vi "rtin_setControlMoveGPIO.vi"(8 "error":errorcluster, 9 "enable":bool=TRUE, 10 "axis":i32, 11 "connection ID":refnum<k5>) -> (0 "error out":errorcluster, 2 "axis_out":i32, 3 "connection ID out":refnum<k5>)   [LabVIEW 2016, in "amc_api.lvlib"]
doc: "This function sets the status for real time input on the selected axis in closed-loop mode."
uses:
  amc_api.lvlib
panel:
  out "jsonRespIn":string
  out "JSON-response":string="{\"jsonrpc\":\"2.0\",\"method\":\"\",\"params\":[5,1.245,true,\"name\"],\"id\":\"1\"}"
  out "JSON request":string
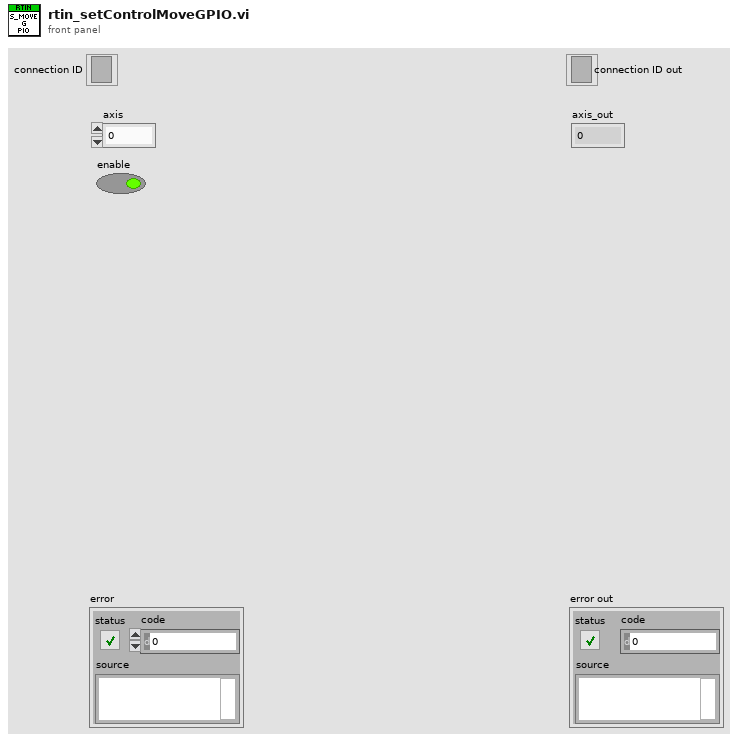
[diagram p1: front panel]
types:
  T1 = cluster{"jsonrpc":string, "method":string, "params":string[], "id":string, "api":i32, "pid":string}
  T2 = enum16{"Standard", "Buffered", "CRLF", "Immediate"}
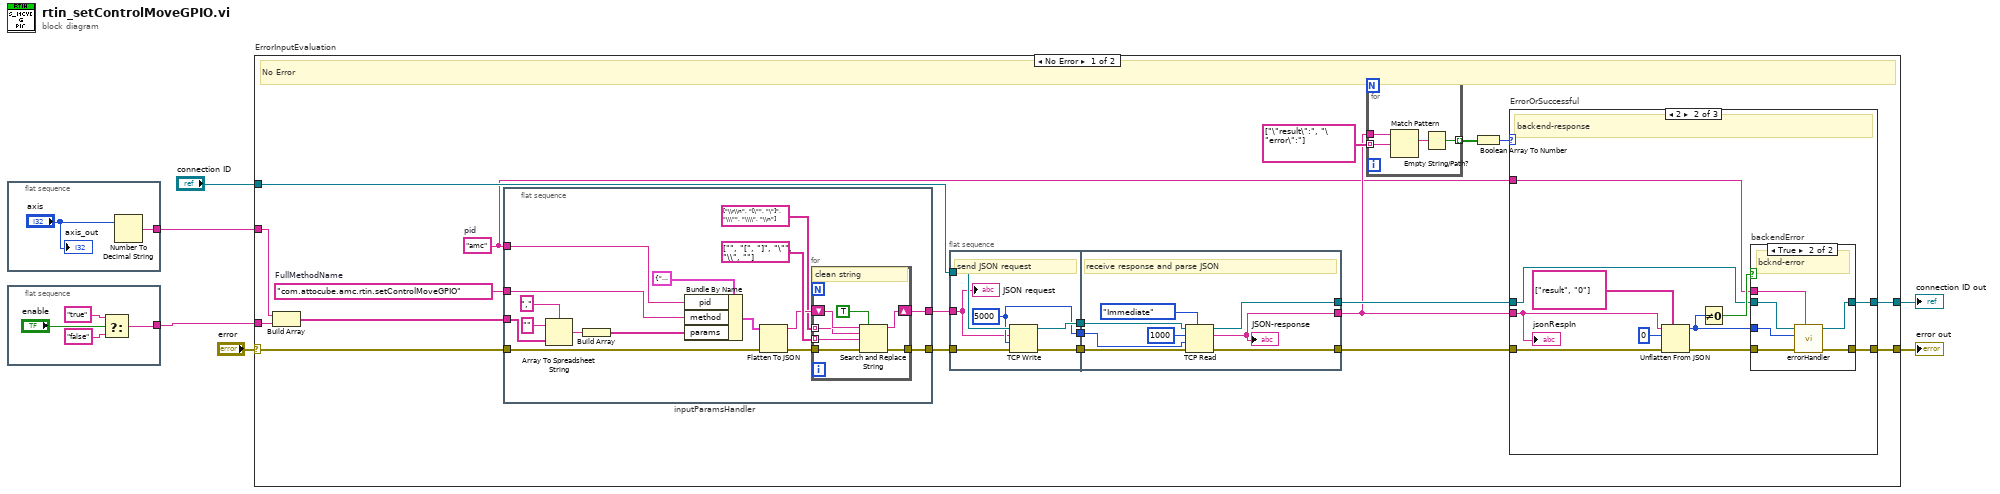
[diagram p0: block diagram]
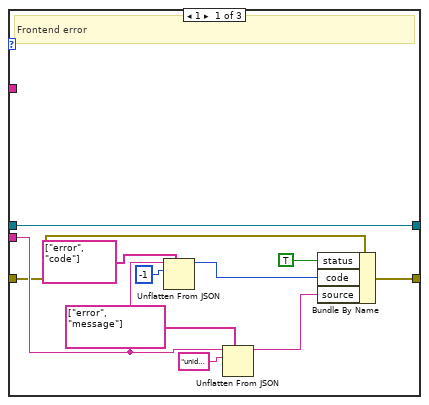
[diagram p2: hidden frame]
diagram:
  n1 = flat-sequence "in_axis" {
    tunnel: [w8] -> w2
    frame #0 {
      n2 = Number To Decimal String(number="axis") -> (decimal integer string=w8:string)  [unwired: 1 in]
      "axis_out" <- "axis"
    }
  }
  n3 = flat-sequence "in_bool" {
    tunnel: [w9] -> w1
    frame #0 {
      n4 = Select(t="true" ("Base"), s="enable", f="false" ("Base")) -> (s? t:f=w9:string)
    }
  }
  n5 = case "ErrorInputEvaluation" shown="No Error" "error" {
    selector: "error" -> [w19 w106]
    tunnel: "connection ID" -> [w29 w107]
    tunnel: [w21 w106] -> w5
    tunnel: [w22 w107] -> w4
    tunnel: w2 -> [w14 _]
    tunnel: w1 -> [w13 _]
    frame No Error {
      w15 = "amc"  # pid
      w20 = "com.attocube.amc.rtin.setControlMoveGPIO"  # FullMethodName
      # "No Error"
      n6 = Build Array ("ParametersArrayString")(w14, w13) -> (w18:string[])
      n7 = flat-sequence "inputParamsHandler" {
        tunnel: [w38] -> w17
        tunnel: w18 -> [w44]
        tunnel: w19 -> [w43]
        tunnel: [w40] -> w16
        tunnel: w20 -> [w34]
        tunnel: w15 -> [w33]
        frame #0 {
          n8 = Array To Spreadsheet String(delimiter (Tab)=",", array=w44, 3:"" ("format string")) -> (spreadsheet string=w46:string)
          n9 = Build Array "Build Array"(w46) -> (w35:string[])
          n10 = Bundle By Name(cluster=T1 {"jsonrpc"="2.0", "method"="com.attocube.amc.res.setRESReadOutFreq", "params"=[], "id"="1", "api"=2, "pid"=""}, "pid"=w33, "method"=w34, "params"=w35) -> (w45:T1)
          n11 = Flatten To JSON(anything=w45, error in (no error)=w43) -> (JSON string=w39:string, 11:w41:errorcluster)  [unwired: 1 in]
          n12 = for {
            tunnel: string[] ["\\r\\n", "[\"", "\"]", "\\\"", "\\\\", "\\n"] ("search string") -> [w52] mode=indexing
            tunnel: string[] ["", "[", "]", "\"", "\\", ""] ("replace string (\"\")") -> [w51] mode=indexing
            shift-right: [w54] -> w38
            shift-left: w39 -> [w53]
            tunnel: w41 -> [w50]
            tunnel: [w49] -> w40
            # "clean string"
            n13 = Search and Replace String(replace all?=TRUE ("replace all? (F)"), input string=w53, search string=w52, replace string=w51, error in=w50) -> (result string=w54:string, error out=w49:errorcluster)  [unwired: 3 in, 2 out]
          }
        }
      }
      n14 = flat-sequence {
        tunnel: w29 -> [w97]
        tunnel: [w95] -> w32
        tunnel: [w96] -> w31
        tunnel: w16 -> [w92]
        tunnel: [w94] -> w30
        tunnel: w17 -> [w93]
        tunnel: [w101] -> w25
        tunnel: w32 -> [w103]
        tunnel: w31 -> [w102]
        tunnel: [w99] -> w24
        tunnel: w30 -> [w100]
        tunnel: [w98] -> w23
        frame #0 {
          w94 = 5000 ("timeout ms (25000)")
          # "send JSON request"
          n15 = TCP Write(connection ID=w97, data in=w93, error in (no error)=w92, 9:w94) -> (connection ID out=w95:refnum<k5>, error out=w96:errorcluster)  [unwired: 1 out]
          "JSON request" <- w93
        }
        frame #1 {
          # "receive response and parse JSON"
          n16 = TCP Read(connection ID=w103, bytes to read=1000, error in (no error)=w102, 7:T2."Immediate" ("mode (standard)"), 9:w100) -> (connection ID out=w101:refnum<k5>, data out=w98:string, error out=w99:errorcluster)
          "JSON-response" <- w98
        }
      }
      n17 = for {
        tunnel: string[] ["\"result\":", "\"error\":"] ("path") -> [w58] mode=indexing
        tunnel: [w56] -> w27 mode=indexing
        tunnel: w23 -> [w59]
        n18 = Match Pattern(string=w59, regular expression=w58) -> (match substring=w57:string)  [unwired: 1 in, 3 out]
        n19 = Empty String/Path?(string/path=w57) -> (empty?=w56:bool)
      }
      n20 = Boolean Array To Number(Boolean array=w27) -> (number=w26:u32)
      n21 = case "ErrorOrSuccessful" shown="2" w26 {
        tunnel: w23 -> [w62 w72 _]
        tunnel: w25 -> [w60 w75 w91]
        tunnel: [w60 w74 w91] -> w22
        tunnel: [w63 w73 w90] -> w21
        tunnel: w24 -> [w61 w76 w90]
        tunnel: w15 -> [_ w71 _]
        frame 1 {
          # "Frontend error"
          n22 = Unflatten From JSON(path=string[] ["error", "code"], JSON string=w62, type and defaults=-1) -> (value=w69:i32)  [unwired: 4 in, 1 out]
          n23 = Unflatten From JSON(path=string[] ["error", "message"], JSON string=w62, type and defaults="unidentified error") -> (value=w70:string)  [unwired: 4 in, 1 out]
          n24 = Bundle By Name(cluster=w61, "status"=TRUE, "code"=w69, "source"=w70) -> (w63:errorcluster)
        }
        frame 2 {
          # "backend-response"
          n25 = Unflatten From JSON(path=string[] ["result", "0"], JSON string=w72, type and defaults=0, error in (no error)=w76) -> (value=w81:i32, error out=w79:errorcluster)  [unwired: 3 in]
          n26 = Not Equal To 0?(x=w81) -> (x != 0?=w80:bool)
          n27 = case "backendError" shown="True" w80 {
            tunnel: w81 -> [_ w89]
            tunnel: w79 -> [w83 w88]
            tunnel: [w82 w87] -> w74
            tunnel: [w83 w86] -> w73
            tunnel: w75 -> [w82 w85]
            tunnel: w71 -> [_ w84]
            frame False {
              # "successful"
            }
            frame True {
              # "bcknd-error"
              n28 = call "errorHandler.vi"("pid"=w84, "error in"=w88, "errNbr"=w89, "connection ID"=w85) -> ("error out 2"=w86:errorcluster, "connection ID out"=w87:refnum<k5>)  [unwired: 6 in]
            }
          }
          "jsonRespIn" <- w72
        }
        frame Default {
          # "NoResponse"
        }
      }
    }
    frame Error {
      # "Error"
    }
  }
  "error out" <- w5
  "connection ID out" <- w4
